vi "Login Details.vi"() -> ()   [LabVIEW 2023]
panel:
  in  "Authority name":string
  out "LOGIN SUCCESS":bool
  in  "Authority":T1
  in  "User Name":string
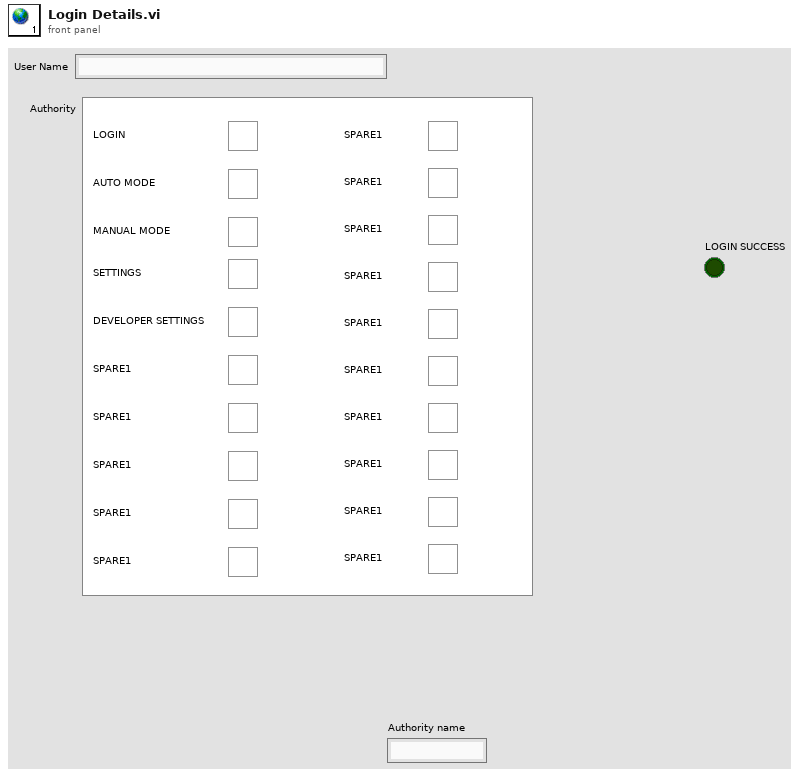
[diagram p1: front panel]
types:
  T1 = cluster{"SCREEN 1":bool, "SCREEN 2":bool, "SCREEN 3":bool, "SCREEN 4":bool, "SCREEN 5":bool, "SCREEN 6":bool, "SCREEN 7":bool, "SCREEN 8":bool, "SCREEN 9":bool, "SCREEN 10":bool, "SCREEN 11":bool, "SCREEN 12":bool, "SCREEN 13":bool, "SCREEN 14":bool, "SCREEN 15":bool, "SCREEN 16":bool, "SCREEN 17":bool, "SCREEN 18":bool, "SCREEN 19":bool, "SCREEN 20":bool}
diagram:
